vi "catchErrors.vi"(8 "error in (no error)":errorcluster, 11 "ScriptListCompiler in":refnum<class "ScriptListCompiler.lvclass">) -> (0 "error out":errorcluster, 2 "error":bool, 3 "ScriptListCompiler out":refnum<class "ScriptListCompiler.lvclass">)   [LabVIEW 2009, in "Compiler.lvlib" / "ScriptListCompiler.lvclass"]
uses:
  ScriptListCompiler.lvclass
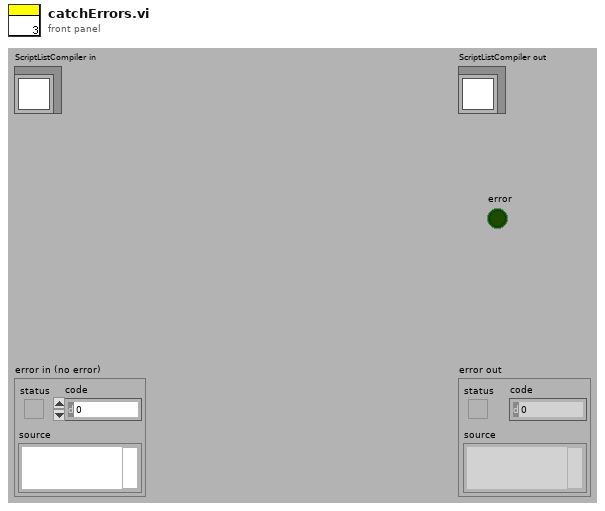
[diagram p1: front panel]
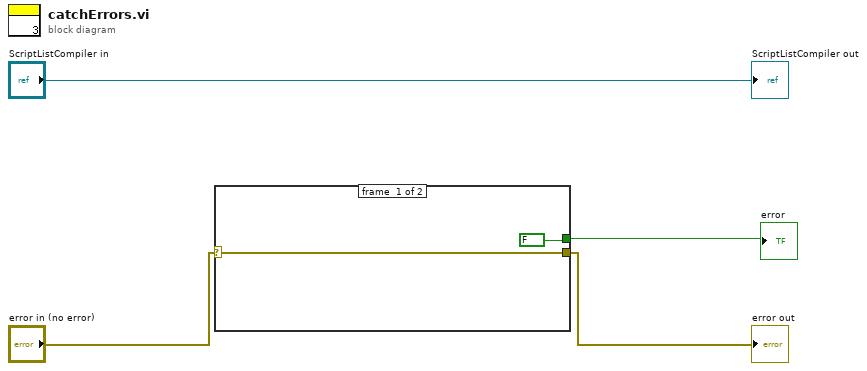
[diagram p0: block diagram]
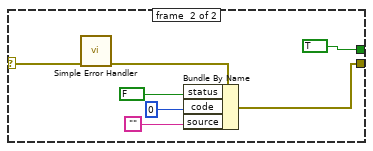
[diagram p2: hidden frame]
diagram:
  n1 = case shown="Error" "error in (no error)" {
    selector: "error in (no error)" -> [w6 w13]
    tunnel: [w6 w8] -> w3
    tunnel: [FALSE TRUE] -> w1
    frame #0 {
    }
    frame #1 {
      n2 = call <vilib>:"Simple Error Handler.vi"("error in (no error)"=w13) -> ("error out"=w12:errorcluster)  [unwired: 4 in, 4 out]
      n3 = Bundle By Name(cluster=w12, "status"=FALSE, "code"=0, "source"="") -> (w8:errorcluster)
    }
  }
  "error out" <- w3
  "error" <- w1
  "ScriptListCompiler out" <- "ScriptListCompiler in"
